vi "Output Protection Status.vi"(8 "error in (no error)":errorcluster, 11 "VISA resource name":refnum<visa-resource-name>) -> (0 "error out":errorcluster, 2 "OVP Tripped":bool, 3 "VISA resource name out":refnum<visa-resource-name>)   [LabVIEW 2021, in "Keithley 2200 Series.lvlib"]
doc: "Sets the OVP state to ON or OFF and returns Over Voltage Protection(OVP) status."
uses:
  <instrlib>/Keithley 2200 Series/Keithley 2200 Series.lvlib
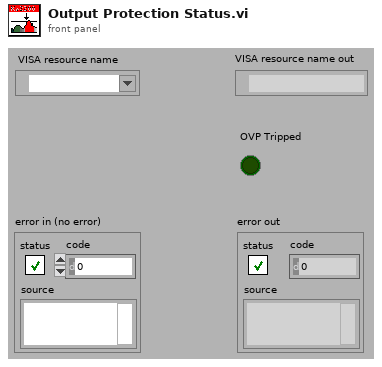
[diagram p1: front panel]
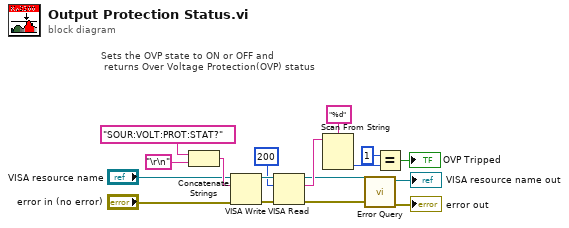
[diagram p0: block diagram]
diagram:
  # "Sets the OVP state to ON or OFF and\n returns Over Voltage Protection(OVP) status"
  n1 = Concatenate Strings("SOUR:VOLT:PROT:STAT?", "\r\n" ("End of Line Constant")) -> (w4:string)
  n2 = VISA Write(VISA resource name="VISA resource name", write buffer=w4, error in (no error)="error in (no error)") -> (VISA resource name out=w16:refnum<visa-resource-name>, error out=w15:errorcluster)  [unwired: 1 out]
  n3 = VISA Read(VISA resource name=w16, byte count=u32 200, error in (no error)=w15) -> (VISA resource name out=w8:refnum<visa-resource-name>, read buffer=w13:string, error out=w7:errorcluster)  [unwired: 1 out]
  n4 = Scan From String(format string="%d", input string=w13) -> (output 1=w11:i32)  [unwired: 2 in, 4 out]
  n5 = call <instrlib>:"Error Query.vi"("error in (no error)"=w7, "VISA resource name"=w8) -> ("error out"=→"error out":errorcluster, "VISA resource name out"=→"VISA resource name out":refnum<visa-resource-name>)  [unwired: 8 out]
  n6 = Equal?(x=1, y=w11) -> (x = y?=→"OVP Tripped":bool)
